vi "Temperature Keysight 34970 MAIN.vi"() -> ()   [LabVIEW 2014]
uses:
  <vilib>/Utility/file.llb/Write To Spreadsheet File (string).vi
panel:
  in  "file path (dialog if empty)":path
  out "time string":string
  out "date string":string
  in  "want seconds? (F)":bool
  in  "date format (0)":enum16{"short", "long", "abbreviated"}(ring)
  out "Waveform Chart":dbl(graph)
  out "Output number":dbl
  in  "stop":bool
  in  "Read delay (in s)":u32=1 min=1 max=60 step=1
  out "Output string":string
  in  "VISA Resource Name":refnum<visa-resource-name>
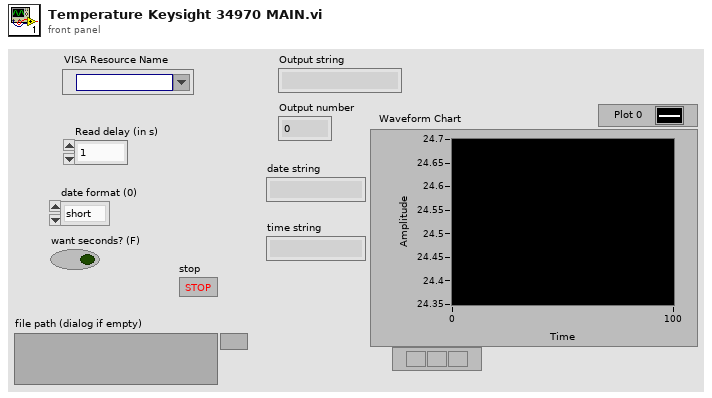
[diagram p1: front panel]
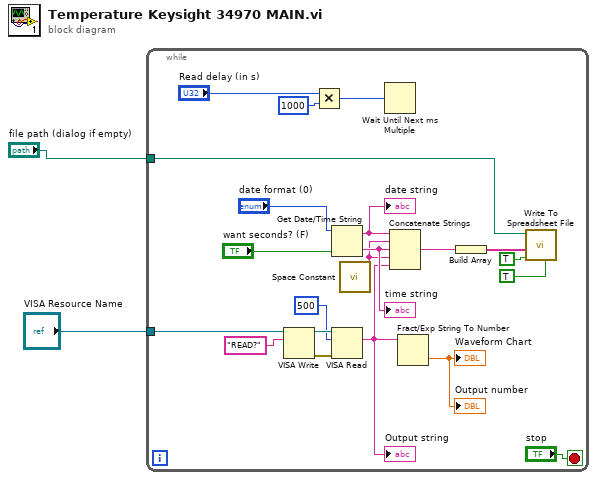
[diagram p0: block diagram]
diagram:
  n1 = while {
    tunnel: "VISA Resource Name" -> [w19]
    tunnel: "file path (dialog if empty)" -> [w3]
    stop <- "stop" stop-if-true
    n2 = VISA Write(VISA resource name=w19, write buffer="READ?") -> (VISA resource name out=w21:refnum<visa-resource-name>, error out=w22:errorcluster)  [unwired: 1 in, 1 out]
    n3 = Multiply(x="Read delay (in s)", y=u32 1000) -> (x*y=w17:u32)
    n4 = Get Date/Time String(date format (0)="date format (0)", want seconds? (F)="want seconds? (F)") -> (date string=w9:string, time string=w6:string)  [unwired: 1 in]
    "date string" <- w9
    "time string" <- w6
    n5 = VISA Read(VISA resource name=w21, byte count=u32 500, error in (no error)=w22) -> (read buffer=w5:string)  [unwired: 3 out]
    "Output string" <- w5
    n6 = call <vilib>:"Space Constant.vi"() -> ("String"=w4:string)
    n7 = Wait Until Next ms Multiple(millisecond multiple=w17) -> ()  [unwired: 1 out]
    n8 = Concatenate Strings(w9, w4, w6, w4, w5) -> (w8:string)
    n9 = Fract/Exp String To Number(string=w5) -> (number=→"Waveform Chart" →"Output number":dbl)  [unwired: 3 in, 1 out]
    n10 = Build Array(w8) -> (w7:string[])
    n11 = call-poly <vilib>:"Write To Spreadsheet File.vi"("transpose? (no:F)"=TRUE, "append to file? (new file:F)"=TRUE, "1D data"=w7, "file path (dialog if empty)"=w3) -> ()  [unwired: 4 in, 1 out]
  }
